vi "Open Parameter.vi"(8 "EN Pop up":bool, 11 "Parameter Path":path) -> (0 "Para Out":dbl[](array[numeric]), 2 "File OK":bool, 3 "dup path":path)   [LabVIEW 2017]
uses:
  <vilib>/Utility/file.llb/Read Delimited Spreadsheet (DBL).vi
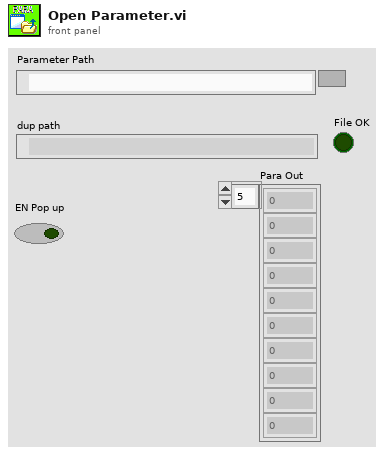
[diagram p1: front panel]
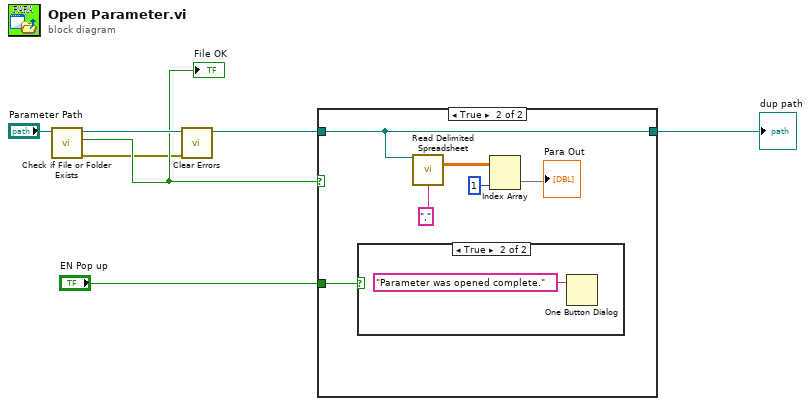
[diagram p0: block diagram]
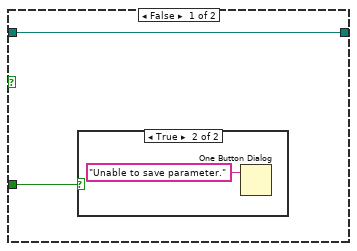
[diagram p2: hidden frame]
diagram:
  n1 = call <vilib>:"Check if File or Folder Exists.vi"("path"="Parameter Path") -> ("error out"=w3:errorcluster, "file or folder exists?"=w5:bool, "dup path"=w6:path)  [unwired: 8 in]
  "File OK" <- w5
  n2 = call <vilib>:"Clear Errors.vi"("error in (no error)"=w3) -> ()  [unwired: 5 in, 2 out]
  n3 = case shown="True" w5 {
    tunnel: w6 -> [w8 w11]
    tunnel: [w8 w11] -> w2
    tunnel: "EN Pop up" -> [w7 w10]
    frame False {
      n4 = case shown="True" w7 {
        frame False {
        }
        frame True {
          n5 = One Button Dialog(message="Unable to save parameter.") -> ()  [unwired: 1 in, 1 out]
        }
      }
    }
    frame True {
      n6 = case shown="True" w10 {
        frame False {
        }
        frame True {
          n7 = One Button Dialog(message="Parameter was opened complete.") -> ()  [unwired: 1 in, 1 out]
        }
      }
      n8 = call-poly <vilib>:"Read Delimited Spreadsheet.vi"("file path (dialog if empty)"=w11, "delimiter (\\t)"="," ("delimiter (\\t)")) -> ("all rows"=w14:dbl[][])  [unwired: 8 in, 5 out]
      n9 = Index Array(array=w14, index (col)=1 ("disabled index (col)")) -> (element=→"Para Out":dbl[])  [unwired: 1 in]
    }
  }
  "dup path" <- w2
